vi "Lectura archivos RPS para análisis version memo.vi"(8 "error in (no error)":errorcluster, 11 "Ruta archivo a analizar":path=path "C:/Users/CIO/Dropbox/cio/Doctores - Trabajos/Dr. Donato Luna Moreno/Codigo Labview/2013/Junio/11Junio/Proyecto [RPS]/data/aire.dat") -> (0 "error out":errorcluster, 2 "Datos(txt)":string, 3 "Tamaño Archivo":i64)   [LabVIEW 2012]
doc: "Este Vi lee archivos de datos del sistema de resonancia de plasmones, extrae la cadena con los datos en ascii y obtiene la información referente a la temperatura inicial y final"
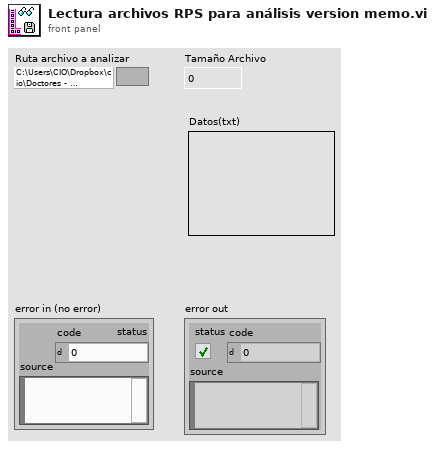
[diagram p1: front panel]
types:
  T1 = enum16{"open", "replace", "create", "open or create", "replace or create", "replace or create with confirmation"}
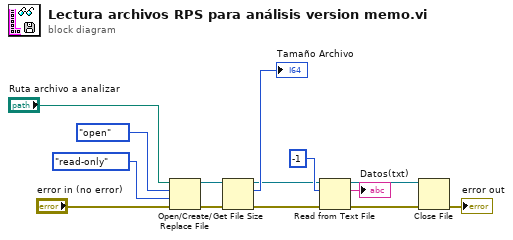
[diagram p0: block diagram]
diagram:
  n1 = Open/Create/Replace File(file path (use dialog)="Ruta archivo a analizar", error in="error in (no error)", operation (0:open)=T1."open", access (0:read/write)=enum16{"read/write", "read-only", "write-only"}."read-only") -> (refnum out=w10:refnum<file>, error out=w9:errorcluster)  [unwired: 2 in, 1 out]
  n2 = Get File Size(file=w10, error in=w9) -> (refnum out=w5:refnum<file>, size (in bytes)=→"Tamaño Archivo":i64, 0:w4:errorcluster)
  n3 = Read from Text File(file (use dialog)=w5, count=-1, error in=w4) -> (refnum out=w3:refnum<file>, text=→"Datos(txt)":string, error out=w2:errorcluster)  [unwired: 1 in, 1 out]
  n4 = Close File(refnum=w3, error in=w2) -> (error out=→"error out":errorcluster)  [unwired: 1 out]
